vi "Fractional-octave Analysis.vi"(0 "scaled signal [EU]":dbl[](array[numeric]) format="%.2f", 1 "averaging type":T5(ring)=enum."Exponential", 2 "averaging parameters":T4={"linear mode"=enum."start averaging once settled", "exponential mode"=enum."Fast", "time constant [ms]"=125.0, "confidence [dB]"=1.0, "peak mode"=enum."start peak detection once settled"} {"confidence [dB]" min=0.01 max=10.0 format="%.2f"; "time constant [ms]" min=0.0 format="%.2f"}, 5 "sampling frequency [Hz]":dbl=10000.0 format="%.2f", 7 "standard":T3, 9 "bandwidth":T2(ring)=enum."1/3 octave", 11 "band number":cluster{"low band":i32, "high band":i32}, 12 "filter init/cont (init:F)":bool, 13 "reset averaging (F)":bool) -> (3 "nominal frequencies (string)":string[](array[string]), 4 "band power [EU^2 rms]":dbl[](array[numeric]) format="%.2f", 6 "nominal frequencies [Hz]":dbl[](array[numeric]) format="%.2f", 8 "settled?":bool, 14 "bandedge frequencies [Hz]":T1(array[cluster]) {"midband" format="%.2f"; "f high" format="%.2f"; "f low" format="%.2f"}, 15 "error":bool)   [LabVIEW 2017]
doc: "Performs a fractional-octave analysis on the input signal.\nThe fractional-octave filters are designed in accordance with one of the following standards:\n ANSI S1.11-1986, Order 3, Type 1-D, optional range;\n Fractional-octave-band filters, class 1, IEC 1260:1995.\nFor both standards, the sampling frequency must be at least 3 times the highest midband frequency for octave analysis and at least 2.5 times the highest midband frequency for 1/3, 1/6, 1/12, or 1/24 octave analysis. Available bandwidths are 1/1, 1/3, 1/6, 1/12, and 1/24 octave.\nThe frequency range is based on the low and high bands specified in the band number cluster. A value of 0 corresponds to the reference frequency of the audio-frequency \nrange 1 kHz. Each successive value corresponds to the next fractional-octave band. Positive values cover the range above 1 kHz, and negative values cover the range below 1 kHz.\nAvailable averaging types are Linear, Exponential (default), Equal confidence, and Peak. Based on the selected averaging type, this VI uses the additional settings in averaging parameters.\nThis VI returns the power in each fractional-octave band.\nTo ensure a continuous filtering operation call this VI the first time with filter init/cont set to FALSE and then call it with filter init/cont set to TRUE."
uses:
  <vilib>/addons/_NISVFA/_Shared subVIs/Controls/svc_Octave Standard.ctl
  <vilib>/addons/Sound and Vibration/svt_Octave/SoundVib_Octave.lvlib
panel:
  # "Linear"
  # "Exponential"
  # "Equal confidence"
  # "Peak"
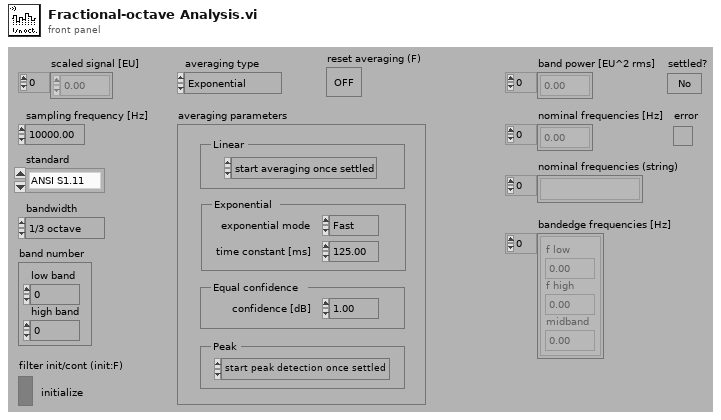
[diagram p1: front panel]
types:
  T1 = cluster{"f low":dbl, "f high":dbl, "midband":dbl}[]
  T2 = enum16{"1 octave", "1/3 octave", "1/6 octave", "1/12 octave", "1/24 octave"}
  T3 = typedef "svc_Octave Standard.ctl" = enum16{"ANSI S1.11", "IEC 61260"}
  T4 = cluster{"linear mode":enum16{"start averaging once settled", "continuous averaging", "single averaging"}, "exponential mode":enum16{"Slow", "Fast", "Impulse", "Custom"}, "time constant [ms]":dbl, "confidence [dB]":dbl, "peak mode":enum16{"start peak detection once settled", "continuous peak detection", "single peak detection"}}
  T5 = enum16{"Linear", "Exponential", "Equal confidence", "Peak"}
  T6 = cluster{"octave filter":cluster{"Octave filter":dbl[]}[], "decimation":i32[], "lowpass filter":dbl[][], "exponential averaging":cluster{"exponential averaging":dbl, "peak detector":dbl}[], "linear averaging":cluster{"squared sum":dbl, "size":dbl}[], "result":dbl[], "# samples since init":u64}
  T7 = cluster{"# special filters":i32, "special filter coefficients":cluster{"filter structure":enum32{"IIR 2nd Order", "IIR 4th Order"}, "Reverse Coefficients":dbl[], "Forward Coefficients":dbl[]}[], "# filters per octave":cluster{"# filters":i32, "starting at":i32}[], "standard filter coefficients":cluster{"filter structure":enum32{"IIR 2nd Order", "IIR 4th Order"}, "Reverse Coefficients":dbl[], "Forward Coefficients":dbl[]}[], "# decimation steps":i32, "lowpass filter coefficients":cluster{"filter structure":enum32{"IIR 2nd Order", "IIR 4th Order"}, "Reverse Coefficients":dbl[], "Forward Coefficients":dbl[]}, "# samples to settle":u64, "special filter bandwidth":dbl[], "standard filter bandwidth":dbl[]}
  T8 = cluster{"octave filter":cluster{"Octave filter":dbl[]}[], "decimation":i32[], "lowpass filter":dbl[][], "exponential averaging":cluster{"exponential averaging":dbl, "peak detector":dbl}[], "linear averaging":cluster{"squared sum":dbl, "size":dbl}[], "result":dbl[], "# samples since init":i32}
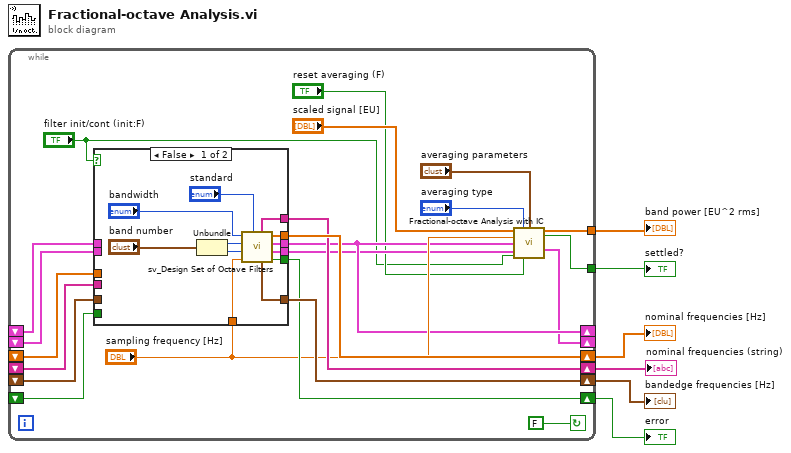
[diagram p0: block diagram]
diagram:
  n1 = while {
    shift-left: _ -> [w19]
    shift-right: [w20] -> w1
    shift-left: _ -> [w21]
    shift-right: [w22] -> w2
    shift-left: _ -> [w23]
    shift-right: [w24] -> w3
    shift-left: _ -> [w25]
    shift-right: [w26] -> w4
    shift-left: _ -> [w28]
    shift-right: [w16] -> _
    shift-left: _ -> [w27]
    shift-right: [w9] -> _
    tunnel: [w10] -> w6
    tunnel: [w11] -> w5
    stop <- FALSE continue-if-true
    n2 = case shown="False" "filter init/cont (init:F)" {
      tunnel: [w35 w46] -> w16
      tunnel: [w34 w45] -> w15
      tunnel: w28 -> [_ w46]
      tunnel: w27 -> [_ w45]
      tunnel: [w33 w44] -> w26
      tunnel: w25 -> [_ w44]
      tunnel: [w32 w43] -> w24
      tunnel: w23 -> [_ w43]
      tunnel: [w31 w42] -> w22
      tunnel: w21 -> [_ w42]
      tunnel: [w30 w41] -> w20
      tunnel: w19 -> [_ w41]
      tunnel: "sampling frequency [Hz]" -> [w29 _]
      frame False {
        n3 = Unbundle("band number") -> ("low band"=w37:i32, "high band"=w36:i32)
        n4 = call <vilib>:"sv_Design Set of Octave Filters.vi"("standard"="standard", "sampling frequency [Hz]"=w29, "high band selector"=w36, "low band selector"=w37, "bandwidth"="bandwidth") -> ("error"=w30:bool, "initialize filter state"=w34:T6, "filter bank parameters"=w35:T7, "nominal frequencies [Hz]"=w33:dbl[], "bandedge frequencies [Hz]"=w31:T1, "nominal frequencies (string)"=w32:string[])  [unwired: 1 in]
      }
      frame True {
      }
    }
    n5 = call <vilib>:"Fractional-octave Analysis with IC.vi"("scaled signal [EU]"="scaled signal [EU]", "averaging type"="averaging type", "averaging parameters"="averaging parameters", "sampling frequency [Hz]"="sampling frequency [Hz]", "filter bank parameters"=w16, "internal filter state IN"=w15, "filter init/cont (init:F)"="filter init/cont (init:F)", "reset averaging (F)"="reset averaging (F)") -> ("band power [EU^2 rms]"=w11:dbl[], "settled?"=w10:bool, "internal filter state OUT"=w9:T8)  [unwired: 5 in]
  }
  "band power [EU^2 rms]" <- w5
  "settled?" <- w6
  "nominal frequencies [Hz]" <- w4
  "nominal frequencies (string)" <- w3
  "bandedge frequencies [Hz]" <- w2
  "error" <- w1
